vi "Read Transmission Data Unit.vi"(8 "error in (no error)":errorcluster, 11 "Network Slave in":refnum<class "Network Slave.lvclass">) -> (0 "error out":errorcluster, 2 "Transmission Data Unit":refnum<class "Transmission Data Unit.lvclass">, 3 "Network Slave out":refnum<class "Network Slave.lvclass">)   [LabVIEW 2021, in "Network Slave.lvclass"]
uses:
  Network Slave.lvclass
  Transmission Data Unit/Transmission Data Unit.lvclass
  Network Slave.lvclass/Network Slave.ctl
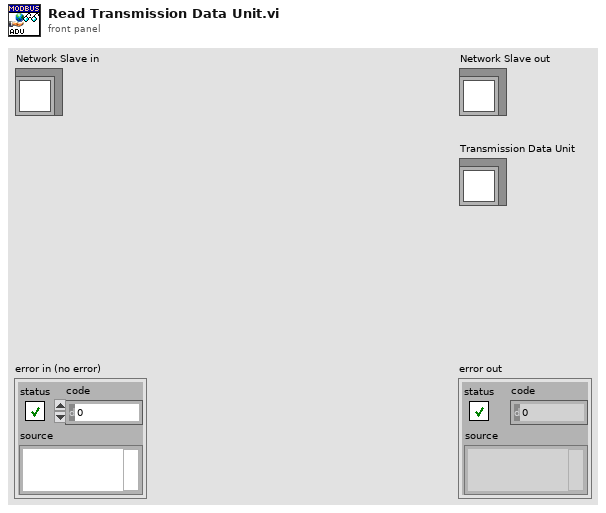
[diagram p1: front panel]
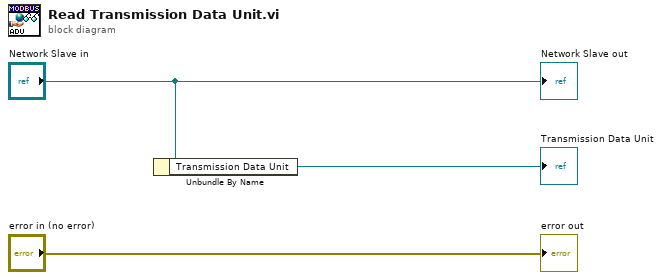
[diagram p0: block diagram]
diagram:
  n1 = Unbundle By Name("Network Slave in") -> ("Transmission Data Unit"=→"Transmission Data Unit":refnum<class "Transmission Data Unit.lvclass">)
  "error out" <- "error in (no error)"
  "Network Slave out" <- "Network Slave in"
